vi "db_advanced_void.vi"(0 "UDL FILEPATH":path, 5 "ERROR IN":errorcluster) -> (14 "SUCCESS?":bool, 19 "LAST QUERY":i32)   [LabVIEW 2018, in "db_lib R3.lvlib"]
uses:
  db_lib R3.lvlib
  <vilib>/addons/database/Connection.llb/DB Tools Open Connec (Path).vi
  <vilib>/addons/database/Connection.llb/Conn Execute.vi
  <vilib>/addons/database/Recordset.llb/Rec Destroy - Connection.vi
  <vilib>/addons/database/NI_Database_API.lvlib
panel:
  in  "QUERIES LIST":string[](array[string])
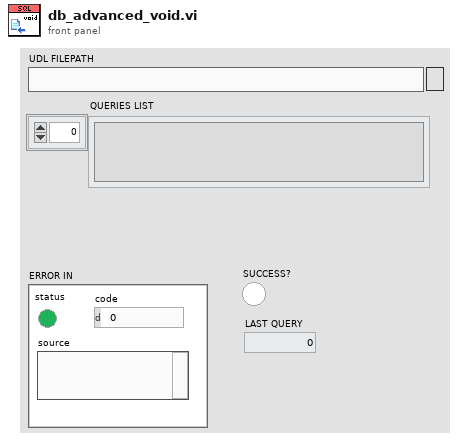
[diagram p1: front panel]
types:
  T1 = typedef "NI_Database_API.lvlib/Conn ObjectReference.ctl" = refnum<k1>
  T2 = typedef "NI_Database_API.lvlib/Rec ObjectReference.ctl" = refnum<k1>
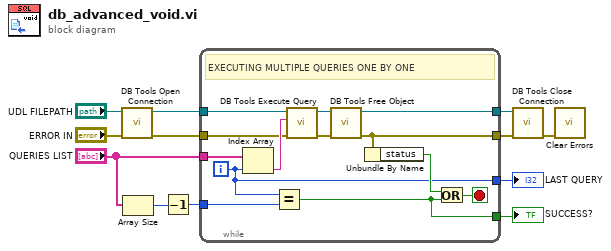
[diagram p0: block diagram]
diagram:
  n1 = call-poly <vilib>:"DB Tools Open Connection.vi"("error in (no error)"="ERROR IN", "connection information"="UDL FILEPATH") -> ("error out"=w9:errorcluster, "connection reference"=w10:T1)  [unwired: 6 in]
  n2 = Array Size(array="QUERIES LIST") -> (size(s)=w7:i32)
  n3 = Decrement(x=w7) -> (x-1=w6:i32)
  n4 = while {
    tunnel: w10 -> [w21]
    tunnel: w9 -> [w20]
    tunnel: "QUERIES LIST" -> [w23]
    tunnel: w6 -> [w19]
    tunnel: [w17] -> w5
    tunnel: [w13] -> w2
    tunnel: [w15] -> w1
    tunnel: [w14] -> w4
    i -> [w15]
    stop <- w18 stop-if-true
    # "EXECUTING MULTIPLE QUERIES ONE BY ONE"
    n5 = Index Array(array=w23, index=w15) -> (element=w22:string)
    n6 = Equal?(x=w15, y=w19) -> (x = y?=w13:bool)
    n7 = call-poly <vilib>:"DB Tools Execute Query.vi"("error in (no error)"=w20, "SQL query"=w22, "connection reference"=w21) -> ("error out"=w25:errorcluster, "recordset reference"=w24:T2)  [unwired: 5 in]
    n8 = call-poly <vilib>:"DB Tools Free Object.vi"("error in (no error)"=w25, "recordset reference"=w24) -> ("error out"=w14:errorcluster, "connection reference"=w17:T1)  [unwired: 8 in]
    n9 = Unbundle By Name(w14) -> ("status"=w16:bool)
    n10 = Or(x=w16, y=w13) -> (x .or. y?=w18:bool)
  }
  "SUCCESS?" <- w2
  "LAST QUERY" <- w1
  n11 = call <vilib>:"DB Tools Close Connection.vi"("error in (no error)"=w4, "connection reference"=w5) -> ("error out"=w3:errorcluster)  [unwired: 5 in]
  n12 = call <vilib>:"Clear Errors.vi"("error in (no error)"=w3) -> ()  [unwired: 5 in, 2 out]
